vi "Save-combined-data.vi"(8 "error in (no error)":errorcluster, 9 "Signal data":dbl[][](array[numeric]), 10 "File path":path) -> (0 "error out":errorcluster)   [LabVIEW 2013, in "MaterialCharacterization.lvlib" / "MC-SM1000.lvclass"]
uses:
  MC-SM1000.lvclass
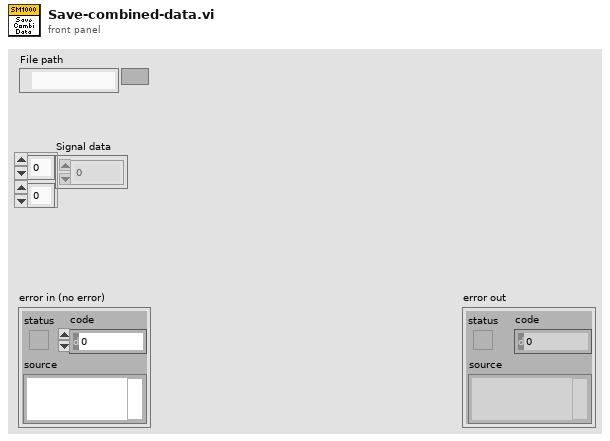
[diagram p1: front panel]
types:
  T1 = enum16{"open", "open or create", "create or replace", "create", "open (read-only)"}
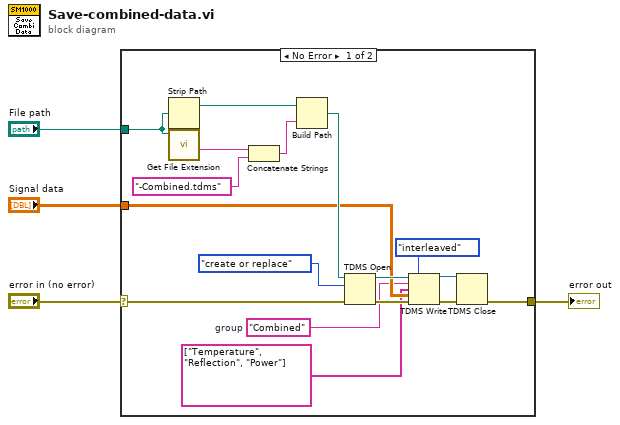
[diagram p0: block diagram]
diagram:
  n1 = case shown="No Error" "error in (no error)" {
    selector: "error in (no error)" -> [w15 w22]
    tunnel: [w6 w22] -> w3
    tunnel: "File path" -> [w19 _]
    tunnel: "Signal data" -> [w12 _]
    frame No Error {
      w11 = "Combined"  # group
      n2 = Strip Path(path=w19) -> (stripped path=w21:path)  [unwired: 1 out]
      n3 = call <vilib>:"Get File Extension.vi"("file"=w19) -> ("filename without extension"=w17:string)  [unwired: 7 in, 3 out]
      n4 = Concatenate Strings(w17, "-Combined.tdms" ("string")) -> (w20:string)
      n5 = Build Path(base path=w21, name or relative path=w20) -> (appended path=w16:path)
      n6 = TDMS Open(8:w15, 10:T1."create or replace" ("operation (0:open)"), 11:w16) -> (0:w13:errorcluster, 3:w14:refnum<k34>)  [unwired: 4 in]
      n7 = TDMS Write(0:w14, 1:enum16{"decimated", "interleaved"}."interleaved" ("data layout (0:decimated)"), 5:w11, 7:string[] ["Temperature", "Reflection", "Power"] ("channel name(s) in (Untitled)"), 9:w12, 11:w13) -> (4:w7:refnum<k34>, 15:w8:errorcluster)  [unwired: 2 out]
      n8 = TDMS Close(8:w8, 11:w7) -> (0:w6:errorcluster)  [unwired: 1 out]
    }
    frame Error {
    }
  }
  "error out" <- w3
